vi "delay_ms.vi"(8 "error in (no error)":errorcluster caption="错误输入（无错误）", 9 "delay time(ms)":i32) -> (0 "error out":errorcluster caption="错误输出")   [LabVIEW 2019]
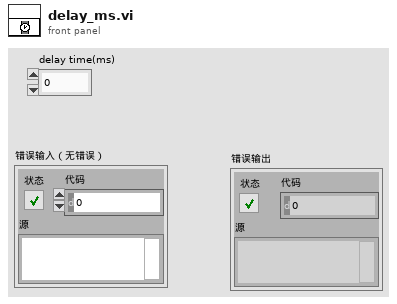
[diagram p1: front panel]
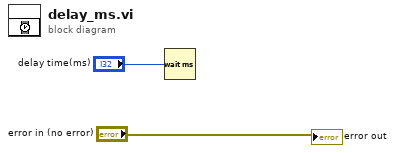
[diagram p0: block diagram]
diagram:
  n1 = Wait (ms)(milliseconds to wait="delay time(ms)") -> ()  [unwired: 1 out]
  "error out" <- "error in (no error)"
